vi "Get DLL Path.vi"(11 "dll name":string) -> (3 "Path":path)   [LabVIEW 2017, in "NI_Robotics_KUKA youBot Host.lvlib"]
uses:
  <vilib>/robotics/KUKA youBot/NI_Robotics_KUKA youBot Host.lvlib
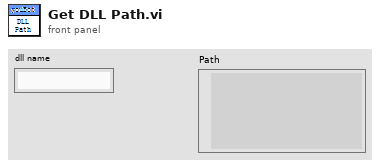
[diagram p1: front panel]
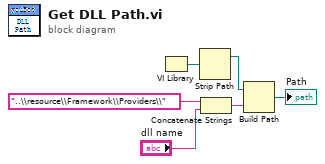
[diagram p0: block diagram]
diagram:
  n1 = VI Library() -> (path=w6:path)
  n2 = Strip Path(path=w6) -> (stripped path=w5:path)  [unwired: 1 out]
  n3 = Concatenate Strings("..\\resource\\Framework\\Providers\\" ("string"), "dll name") -> (w2:string)
  n4 = Build Path(base path=w5, name or relative path=w2) -> (appended path=→"Path":path)
